vi "Simulation.vi"() -> ()   [LabVIEW 2023]
uses:
  <vilib>/addons/Modulation/Digital/General/MT Generate Bits (Galois, PN Order).vi
  <vilib>/addons/Modulation/Digital/Support/Common/Validators/mod_Generate Bits Validate.vi
  <vilib>/addons/Modulation/Analog/support/mod_Set Error Source.vi
  <vilib>/addons/Modulation/Digital/Support/Common/Validators/mod_AWGN Validate.vi
  <vilib>/addons/Modulation/Digital/Impairments/subVIs/mod_createSeeds.vi
  <vilib>/addons/Modulation/Analog/support/Validators/mod_Fractional Resample Validate.vi
  <vilib>/addons/Modulation/Analog/support/Validators/mod_Check Flush State.vi
  <vilib>/addons/Modulation/Analog/support/mod_FractionalResampler.vi
  <vilib>/addons/Modulation/Analog/support/mod_Integer Rate Interpolation.vi
  <vilib>/addons/Modulation/Digital/Support/Common/Validators/mod_Validate Samples Per Symbol.vi
  <vilib>/addons/Modulation/Analog/support/Validators/mod_Validate Complex Waveform.vi
  <vilib>/addons/Modulation/Analog/support/mod_PerformResampling.vi
  <vilib>/addons/Modulation/Analog/support/Validators/mod_WFErrorHandler.vi
  <vilib>/addons/Modulation/Digital/General/subVIs/mod_Generate Bits PN Sequence.vi
  <vilib>/addons/Modulation/Digital/General/MT Generate MSK System Parameters.vi
  <vilib>/addons/Modulation/Digital/Support/Common/Validators/mod_Generate Filter Coefficients Validate.vi
  <vilib>/addons/Modulation/Digital/General/subVIs/mod_Generate Filter Coefficients.vi
  <vilib>/Analysis/1siggen.llb/Gaussian White Noise (obs 90).vi
  <vilib>/Utility/error.llb/Error Cluster From Error Code.vi
  <vilib>/addons/Modulation/Analog/support/mod_Resampling Factors.vi
  <vilib>/addons/Modulation/Analog/support/mod_ResamplingFilter.vi
  <vilib>/addons/Modulation/Analog/support/mod_Generate Integer Interpolation Filter.vi
  <vilib>/addons/Modulation/niDMT.lvlib
  <vilib>/addons/Modulation/niAMT.lvlib
panel:
  in  "filter length (symbols) 2":i32=8
  in  "filter length (symbols)":i32=8
  in  "Eb/N0 (10 dB)":dbl=10.0 format="%.2f"
  out "Demodulation constaltion":T1(graph)
  out "error out 2":errorcluster
  in  "symbol rate (Hz) 2":dbl=1.0 caption="symbol rate (Hz)" format="%.2f"
  in  "error in (no error) 2":errorcluster
  out "error out":errorcluster
  in  "error in (no error)":errorcluster
  out "inputSeq":dbl[](graph)
  out "modulation constaltion":T1(graph)
  out "demodulation":i8[](graph)
  in  "symbol rate (Hz)":dbl=1.0 format="%.2f"
  out "modulation":dbl[](graph)
  out "filter shape":dbl[](graph)
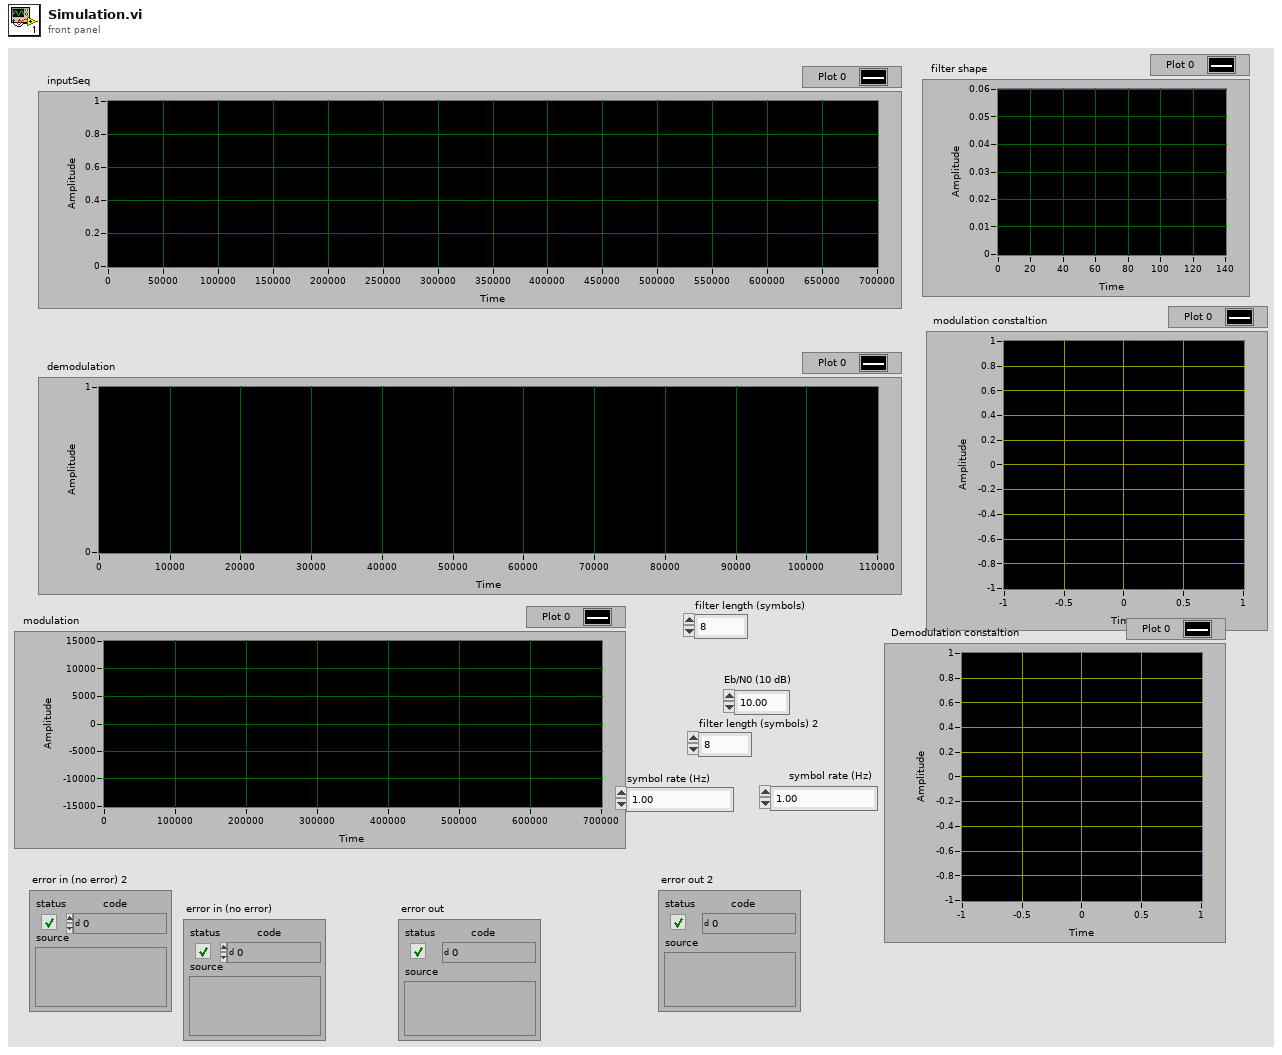
[diagram p1: front panel]
types:
  T1 = cluster{"constellation":dbl[], "oversampled data":dbl[]}[]
  T2 = enum16{"none", "Raised Cosine", "Root Raised Cos", "Gaussian"}
  T3 = enum16{"FSK", "PSK", "QAM", "MSK", "PAM", "ASK", "CPM"}
  T4 = cluster{"differential encoding enable":enum16{"disable", "enable"}, "samples per symbol (16)":i32}
  T5 = typedef "niAMT.lvlib/Complex Data Waveform.ctl" = cluster{"t0":dbl, "dt":dbl, "Y":cdb[]}
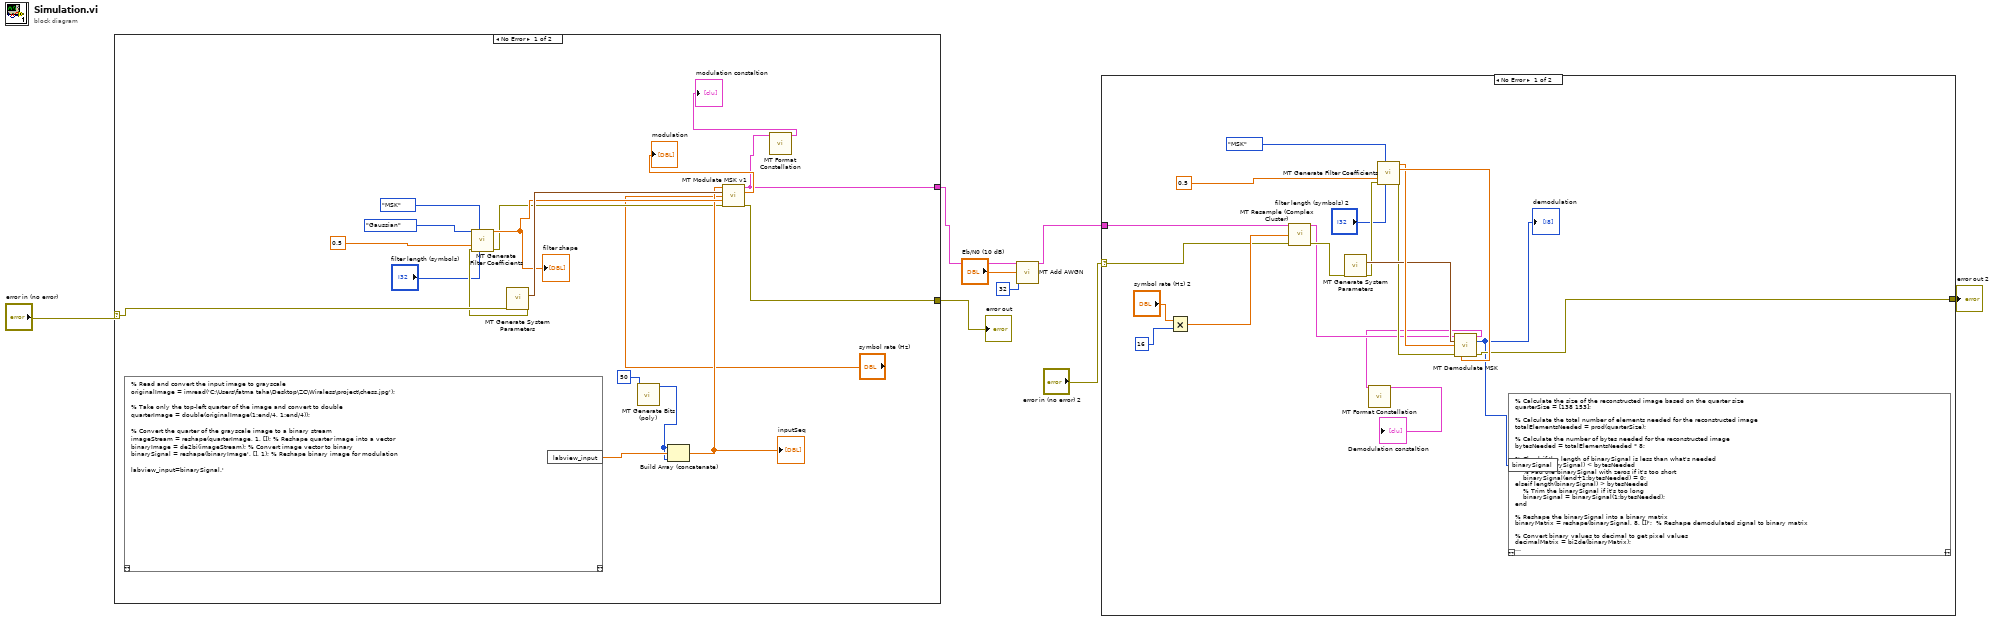
[diagram p0: block diagram]
diagram:
  n1 = case shown="No Error" "error in (no error)" {
    selector: "error in (no error)" -> [w18 w27]
    tunnel: [w15 w27] -> w7
    tunnel: [w14 _] -> w4
    frame No Error {
      n2 = script code="% Read and convert the input image to grayscale\noriginalImage = imread('C:\\Users\\fatma taha\\Desktop\\ZC\\Wiraless\\project\\chess.jpg');\n\n% Take only the top-left quarter of the image and convert to double\nquarterImage = double(originalImage(1:end/4, 1:end/4));\n\n% Convert the quarter of the grayscale image to a binary stream\nimageStream = reshape(quarterImage, 1, []); % Reshape quarter image into a vector\nbinaryImage = de2bi(imageStream); % Convert image vector to binary\nbinarySignal = reshape(binaryImage', [], 1); % Reshape binary image for modulation\n\nlabview_input=binarySignal.'"() -> ("labview_input"=w11:dbl[])  [unwired: 1 in, 1 out]
      n3 = call-poly <vilib>:"MT Generate System Parameters.vi"("error in (no error)"=w18) -> ("MSK system parameters"=w23:T4, "error out"=w17:errorcluster)  [unwired: 12 in, 1 out]
      n4 = call <vilib>:"MT Generate Filter Coefficients.vi"("pulse shaping filter (none)"=T2."Gaussian", "modulation type"=T3."MSK", "filter parameter"=0.5, "error in (no error)"=w17, "filter length (symbols)"="filter length (symbols)") -> ("pulse shaping filter coefficients"=w22:dbl[], "error out"=w16:errorcluster)  [unwired: 8 in, 1 out]
      "filter shape" <- w22
      n5 = call-poly <vilib>:"MT Generate Bits (poly).vi"("total bits (128)"=50) -> ("output bit stream"=w9:i8[])  [unwired: 12 in, 2 out]
      n6 = Build Array (concatenate)(w9, w11, w9) -> (w20:dbl[])
      "inputSeq" <- w20
      n7 = call <vilib>:"MT Modulate MSK v1.vi"("input bit stream"=w20, "MSK system parameters"=w23, "symbol rate (Hz)"="symbol rate (Hz)", "pulse shaping filter coefficients"=w22, "error in (no error)"=w16) -> ("output complex waveform"=w14:T5, "symbols out"=→"modulation":dbl[], "error out"=w15:errorcluster)  [unwired: 8 in]
      n8 = call <vilib>:"MT Format Constellation.vi"("waveform"=w14) -> ("constellation graph"=→"modulation constaltion":T1)  [unwired: 13 in, 1 out]
    }
    frame Error {
    }
  }
  "error out" <- w7
  n9 = call <vilib>:"MT Add AWGN.vi"("input complex waveform"=w4, "bits per symbol (1)"=32, "Eb/N0 (10 dB)"="Eb/N0 (10 dB)") -> ("output complex waveform"=w3:T5)  [unwired: 10 in, 2 out]
  n10 = case shown="No Error" "error in (no error) 2" {
    selector: "error in (no error) 2" -> [w38 w47]
    tunnel: [w34 w47] -> w5
    tunnel: w3 -> [w29 _]
    frame No Error {
      n11 = Multiply(x="symbol rate (Hz) 2", y=16 ("samples per symbol (16)")) -> (x*y=w41:dbl)
      n12 = call <vilib>:"MT Resample (Complex Cluster).vi"("input complex waveform"=w29, "desired sample rate (Hz)"=w41, "error in (no error)"=w38) -> ("output complex waveform"=w32:T5, "error out"=w37:errorcluster)  [unwired: 11 in]
      n13 = call-poly <vilib>:"MT Generate System Parameters.vi"("error in (no error)"=w37) -> ("MSK system parameters"=w42:T4, "error out"=w36:errorcluster)  [unwired: 12 in, 1 out]
      n14 = call <vilib>:"MT Generate Filter Coefficients.vi"("modulation type"=T3."MSK", "filter parameter"=0.5, "error in (no error)"=w36, "filter length (symbols)"="filter length (symbols) 2") -> ("pulse shaping filter coefficients"=w43:dbl[], "matched filter coefficients"=w44:dbl[], "error out"=w35:errorcluster)  [unwired: 9 in]
      n15 = call <vilib>:"MT Demodulate MSK.vi"("input complex waveform"=w32, "MSK system parameters"=w42, "matched filter coefficients"=w43, "error in (no error)"=w35, "pulse shaping filter coefficients"=w44) -> ("recovered complex waveform"=w31:T5, "output bit stream"=w33:i8[], "error out"=w34:errorcluster)  [unwired: 5 in, 3 out]
      "demodulation" <- w33
      n16 = call <vilib>:"MT Format Constellation.vi"("waveform"=w31) -> ("constellation graph"=→"Demodulation constaltion":T1)  [unwired: 13 in, 1 out]
      n17 = script code="% Calculate the size of the reconstructed image based on the quarter size\nquarterSize = [138 153];\n\n% Calculate the total number of elements needed for the reconstructed image\ntotalElementsNeeded = prod(quarterSize);\n\n% Calculate the number of bytes needed for the reconstructed image\nbytesNeeded = totalElementsNeeded * 8;\n\n% Check if the length of binarySignal is less than what's needed\nif length(binarySignal) < bytesNeeded\n    % Pad the binarySignal with zeros if it's too short\n    binarySignal(end+1:bytesNeeded) = 0;\nelseif length(binarySignal) > bytesNeeded\n    % Trim the binarySignal if it's too long\n    binarySignal = binarySignal(1:bytesNeeded);\nend\n\n% Reshape the binarySignal into a binary matrix\nbinaryMatrix = reshape(binarySignal, 8, [])';  % Reshape demodulated signal to binary matrix\n\n% Convert binary values to decimal to get pixel values\ndecimalMatrix = bi2de(binaryMatrix);  \n\n% Normalize the pixel values to the range [0, 255]\nminVal = double(min(decimalMatrix));\nmaxVal = double(max(decimalMatrix));\nnormalizedDecimalMatrix = (double(decimalMatrix) - minVal) / (maxVal - minVal) * 255;\n\n% Reshape normalized decimal matrix to quarter image size\n% Ensure the total number of elements matches the required size\nreconstructedImage = reshape(normalizedDecimalMatrix(1:totalElementsNeeded), quarterSize);\n\n% Convert to uint8 for image display\nreconstructedQuarterImage = uint8(reconstructedImage);\n\n% Save the reconstructed quarter image\nimwrite(reconstructedQuarterImage, 'C:\\Users\\fatma taha\\Desktop\\ZC\\Wiraless\\project\\reconstructed_image_labview.png');"("binarySignal"=w33) -> ()  [unwired: 1 in, 1 out]
    }
    frame Error {
    }
  }
  "error out 2" <- w5
